vi "niRFUtil RFHS Channelizer BufferLen CSG.vi"(0 "Buffer":csg[](array[numeric])) -> (4 "Length":i32)   [LabVIEW 2015, in "niRFUtil.lvlib"]
uses:
  niRFUtil.lvlib
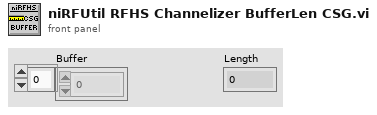
[diagram p1: front panel]
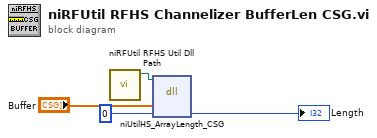
[diagram p0: block diagram]
diagram:
  n1 = call "niRFUtil RFHS Util Dll Path.vi"() -> ("Path"=w3:path)  [unwired: 7 in, 4 out]
  n2 = dll-call lib="?" fn="niUtilHS_ArrayLength_CSG"(path in=w3, "buf"="Buffer", "length"=0) -> ("length"=→"Length":i32)  [unwired: 4 in, 2 out]
